vi "Set Label Config.vi"(8 "error in (no error)":errorcluster, 11 "RT Data in":T1 {"Label Transfer Config"."Block Data Refs"."Data Reference" format="%.0x"; "Status Config"."HWOut Dur Ref" format="%.0x"; "Status Config"."HWIn Dur Ref" format="%.0x"; "Status Config"."Error Data Ref" format="%.0x"; "HWOutput Channels"."Labels Settings"."Label" format="%.0o"; "HWInput Channels"."Labels Settings"."Label" format="%.0o"}) -> (0 "error out":errorcluster, 3 "RT Data out":T1 {"Label Transfer Config"."Block Data Refs"."Data Reference" format="%.0x"; "Status Config"."HWOut Dur Ref" format="%.0x"; "Status Config"."HWIn Dur Ref" format="%.0x"; "Status Config"."Error Data Ref" format="%.0x"; "HWOutput Channels"."Labels Settings"."Label" format="%.0o"; "HWInput Channels"."Labels Settings"."Label" format="%.0o"})   [LabVIEW 2015, in "AIT 429 Engine.lvlib"]
uses:
  AIT 429 Engine.lvlib
  RT Controls/RT Data.ctl
  RT Controls/RT HW Channel.ctl
  RT Controls/RT Label Settings.ctl
  Shared/Controls and Global/Label.ctl
  Shared/Controls and Global/transferPeriod.ctl
  RT Controls/Driver Data.ctl
  RT Controls/RT Word Settings.ctl
  <vilib>/NI Veristand/Custom Device API/Block Data Reference.ctl
  <vilib>/NI Veristand/Custom Device API/Data Reference.ctl
  RT Controls/RT Param Setting.ctl
  Shared/Controls and Global/Start Bit.ctl
  Shared/Controls and Global/Number of Bits.ctl
  Shared/Controls and Global/TransferType.ctl
  RT Controls/Error Qs.ctl
  RT Controls/Status Channels Config.ctl
  RT Controls/FIFO.ctl
  RT Controls/Label Transfer Config.ctl
  <instrlib>/AIT 429/AIT 429.lvlib
  Shared/AIT 429 Shared.lvlib
  <vilib>/NI Veristand/Custom Device API/Custom Device API.lvlib
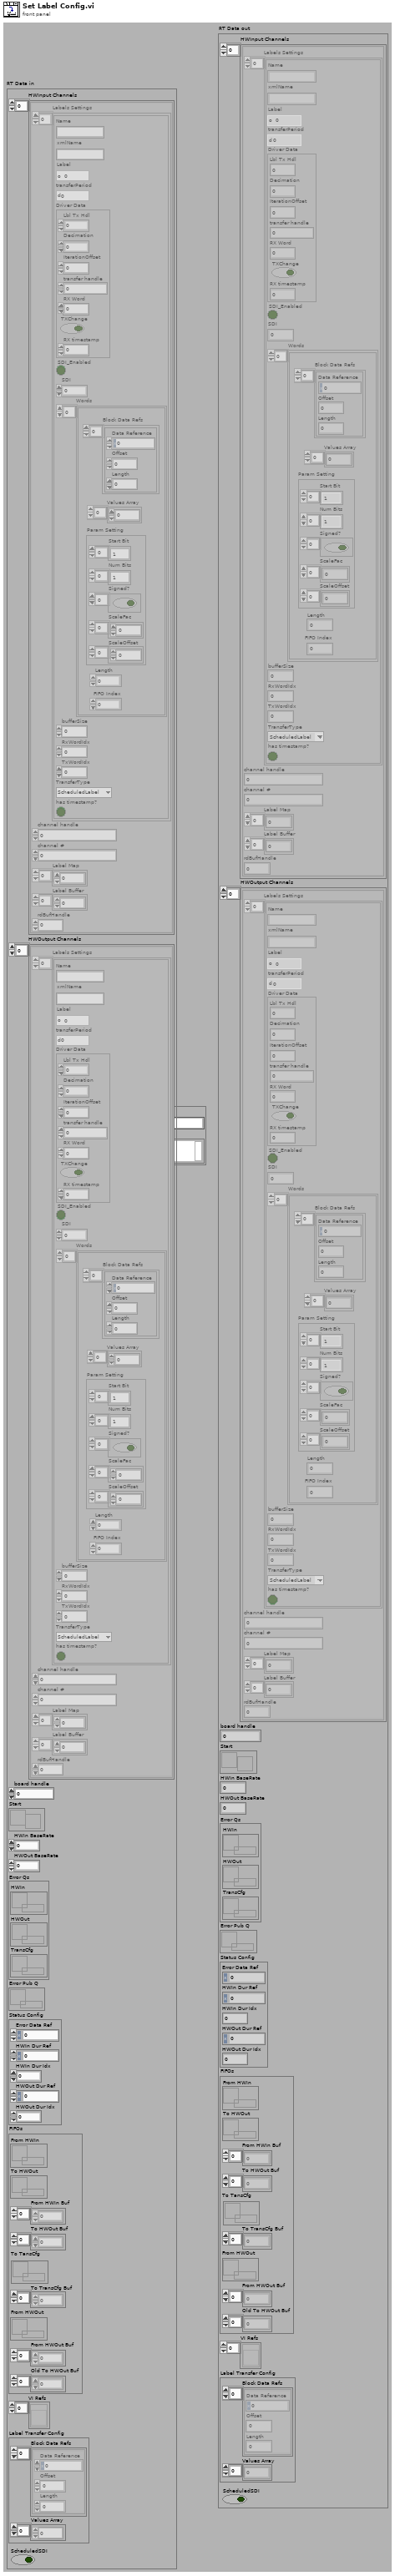
[diagram p1: front panel]
types:
  T1 = typedef "AIT 429 Engine.lvlib/RT Data.ctl" = cluster{"HWInput Channels":T2[], "HWOutput Channels":T2[], "board handle":u32, "Start":refnum<notifier>, "HWIn BaseRate":i64, "HWOut BaseRate":i64, "Error Qs":T14, "Error Pub Q":refnum<queue>, "Status Config":T15, "FIFOs":T16, "VI Refs":refnum<vi>[], "Label Transfer Config":T17, "ScheduledSDI":bool}
  T2 = typedef "AIT 429 Engine.lvlib/RT HW Channel.ctl" = cluster{"Labels Settings":T3[], "channel handle":u32, "channel #":u16, "Label Map":i32[], "Label Buffer":u32[], "rdBufHandle":u32}
  T3 = typedef "AIT 429 Engine.lvlib/RT Label Settings.ctl" = cluster{"Name":string, "xmlName":string, "Label":T4, "transferPeriod":T5, "Driver Data":T6, "SDI_Enabled":bool, "SDI":u8, "Words":T7[], "bufferSize":u32, "RxWordIdx":i32, "TxWordIdx":i32, "TransferType":T13, "has timestamp?":bool}
  T4 = typedef "AIT 429 Shared.lvlib/Label.ctl" = u8
  T5 = typedef "AIT 429 Shared.lvlib/transferPeriod.ctl" = u32
  T6 = typedef "AIT 429 Engine.lvlib/Driver Data.ctl" = cluster{"Lbl Tx Hdl":u32, "Decimation":i32, "IterationOffset":i32, "transfer handle":u32, "RX Word":u32, "TXChange":bool, "RX timestamp":dbl}
  T7 = typedef "AIT 429 Engine.lvlib/RT Word Settings.ctl" = cluster{"Block Data Refs":T8[], "Values Array":dbl[], "Length":i32, "FIFO Index":i32, "Param Setting":T10}
  T8 = typedef "Custom Device API.lvlib/Block Data Reference.ctl" = cluster{"Data Reference":T9, "Offset":u64, "Length":u64}
  T9 = typedef "Custom Device API.lvlib/Data Reference.ctl" = i32
  T10 = typedef "AIT 429 Engine.lvlib/RT Param Setting.ctl" = cluster{"Start Bit":T11[], "Num Bits":T12[], "Signed?":bool[], "ScaleFac":dbl[], "ScaleOffset":dbl[]}
  T11 = typedef "AIT 429 Shared.lvlib/Start Bit.ctl" = i32
  T12 = typedef "AIT 429 Shared.lvlib/Number of Bits.ctl" = i32
  T13 = typedef "AIT 429 Shared.lvlib/TransferType.ctl" = enum16{"ScheduledLabel", "Acyclic", "Block", "Strobe"}
  T14 = typedef "AIT 429 Engine.lvlib/Error Qs.ctl" = cluster{"HWIn":refnum<queue>, "HWOut":refnum<queue>, "TransCfg":refnum<queue>}
  T15 = typedef "AIT 429 Engine.lvlib/Status Channels Config.ctl" = cluster{"Error Data Ref":T9, "HWIn Dur Ref":T9, "HWIn Dur Idx":i32, "HWOut Dur Ref":T9, "HWOut Dur Idx":i32}
  T16 = typedef "AIT 429 Engine.lvlib/FIFO.ctl" = cluster{"From HWIn":refnum<k33>, "To HWOut":refnum<k33>, "From HWIn Buf":dbl[], "To HWOut Buf":dbl[], "To TansCfg":refnum<k33>, "To TransCfg Buf":dbl[], "From HWOut":refnum<k33>, "From HWOut Buf":dbl[], "Old To HWOut Buf":dbl[]}
  T17 = typedef "AIT 429 Engine.lvlib/Label Transfer Config.ctl" = cluster{"Block Data Refs":T8[], "Values Array":dbl[]}
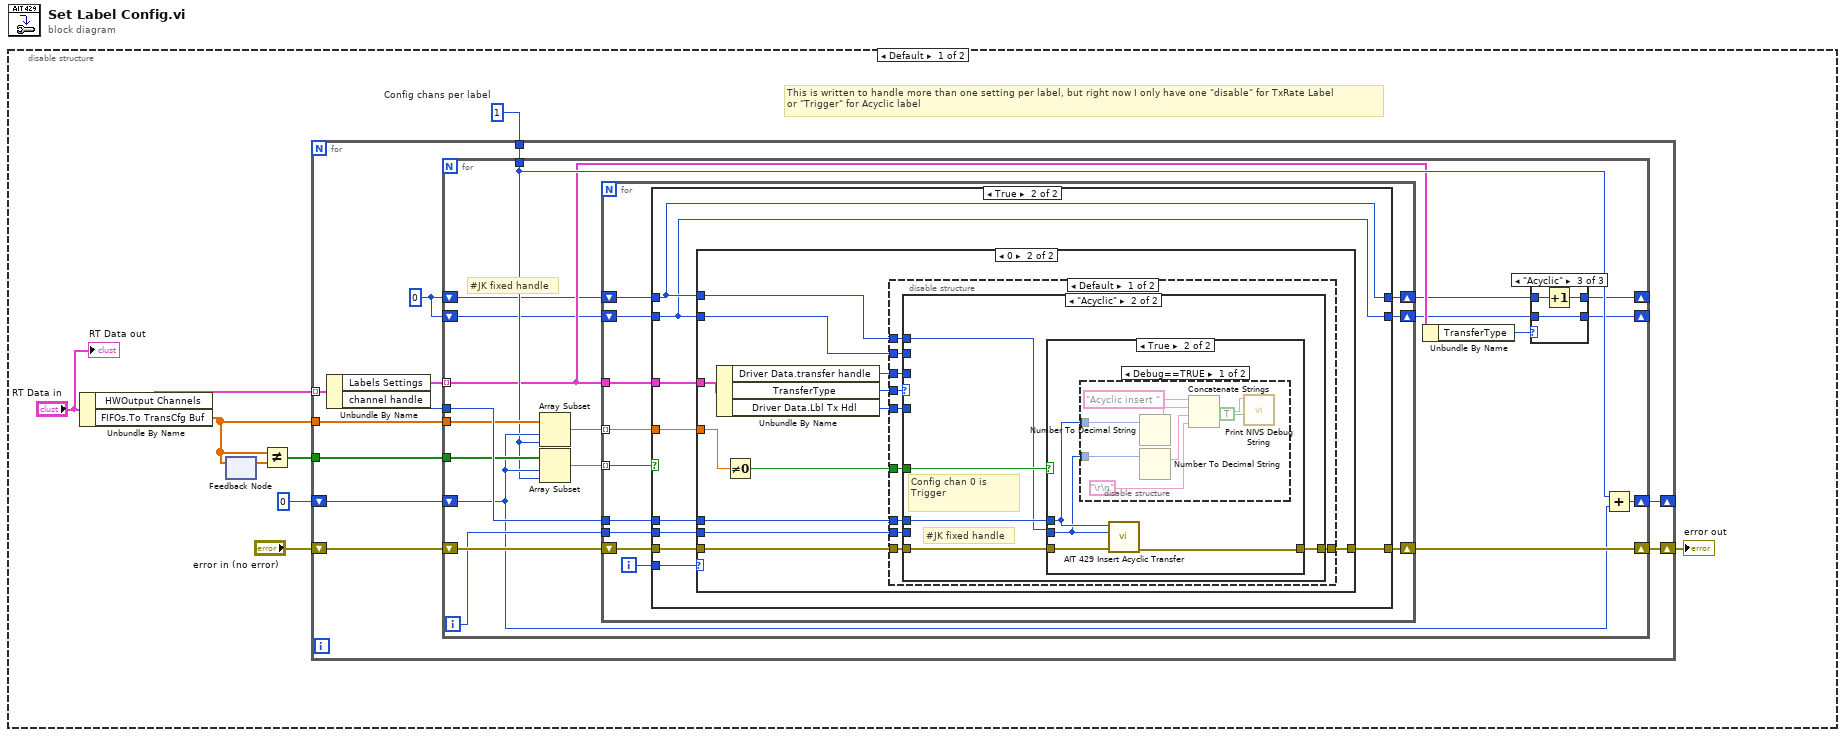
[diagram p0: block diagram]
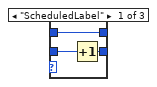
[diagram p2: hidden frame]
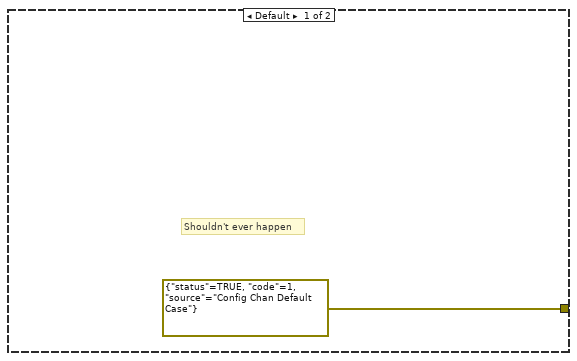
[diagram p5: hidden frame]
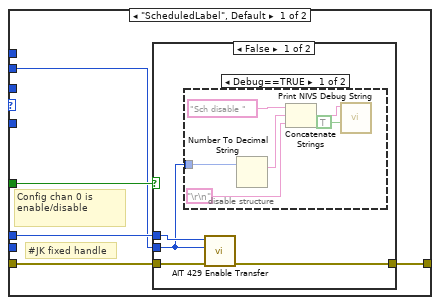
[diagram p6: hidden frame]
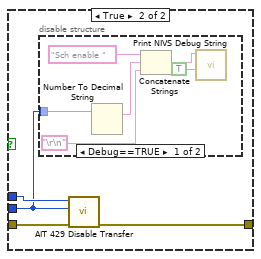
[diagram p8: hidden frame]
diagram:
  n1 = disable-structure shown="Default" {
    frame condition #0 (active) {
      w2 = 1  # Config chans per label
      # "This is written to handle more than one setting per label, but right now I only have one \"disable\" for TxRate Label \nor \"Trigger\" for Acyclic label"
      n2 = Unbundle By Name("RT Data in") -> ("HWOutput Channels"=w7:T2[], "FIFOs.To TransCfg Buf"=w1:dbl[])
      n3 = feedback #1() -> (w5:dbl[])  [unwired: 1 in]
      n4 = feedback-in #1(w1) -> ()
      n5 = Not Equal?(x=w1, y=w5) -> (x != y?=w4:bool[])
      n6 = for {
        shift-right: [w19] -> w8
        shift-left: "error in (no error)" -> [w20]
        tunnel: w7 -> [w18] mode=indexing
        shift-right: [w12] -> _
        shift-left: 0 ("index") -> [w14]
        tunnel: w4 -> [w15]
        tunnel: w2 -> [w13]
        tunnel: w1 -> [w11]
        w10 = u32 0 ("Lbl Tx Hdl")
        n7 = Unbundle By Name(w18) -> ("Labels Settings"=w17:T3[], "channel handle"=w16:u32)
        n8 = for {
          tunnel: w17 -> [w25] mode=indexing
          tunnel: w16 -> [w37]
          shift-right: [w38] -> w19
          shift-left: w20 -> [w39]
          tunnel: w15 -> [w36]
          tunnel: w13 -> [w30]
          shift-right: [w34] -> w12
          shift-left: w14 -> [w31]
          tunnel: w11 -> [w32]
          shift-right: [w27] -> _
          shift-left: w10 -> [w22]
          shift-right: [w26] -> _
          shift-left: w10 -> [w21]
          i -> [w33]
          # "#JK fixed handle"
          n9 = Array Subset(array=w32, index=w31, length=w30) -> (w29:dbl[])
          n10 = Array Subset(array=w36, index=w31, length=w30) -> (w35:bool[])
          n11 = for {
            tunnel: w37 -> [w57]
            tunnel: w35 -> [w55] mode=indexing
            tunnel: w33 -> [w56]
            shift-right: [w58] -> w38
            shift-left: w39 -> [w59]
            tunnel: w29 -> [w54] mode=indexing
            tunnel: w25 -> [w50]
            shift-right: [w51] -> w23
            shift-left: w21 -> [w48]
            shift-right: [w52] -> w24
            shift-left: w22 -> [w49]
            i -> [w53]
            n12 = case shown="True" w55 {
              tunnel: w59 -> [w62 w71]
              tunnel: [w62 w70] -> w58
              tunnel: w57 -> [_ w69]
              tunnel: w56 -> [_ w68]
              tunnel: w54 -> [_ w66]
              tunnel: w53 -> [_ w67]
              tunnel: w50 -> [_ w65]
              tunnel: [w61 w64] -> w52
              tunnel: [w60 w63] -> w51
              tunnel: w49 -> [w61 w64]
              tunnel: w48 -> [w60 w63]
              frame False {
              }
              frame True {
                n13 = case shown="0" w67 {
                  tunnel: w71 -> [_ w84]
                  tunnel: [errorcluster {"status"=TRUE, "code"=1, "source"="Config Chan Default Case"} ("error out") w83] -> w70
                  tunnel: w69 -> [_ w82]
                  tunnel: w68 -> [_ w81]
                  tunnel: w66 -> [_ w80]
                  tunnel: w65 -> [_ w78]
                  tunnel: w64 -> [_ w74]
                  tunnel: w63 -> [_ w73]
                  frame Default {
                    # "Shouldn't ever happen"
                  }
                  frame 0 {
                    n14 = Unbundle By Name(w78) -> ("Driver Data.transfer handle"=w76:u32, "TransferType"=w77:T13, "Driver Data.Lbl Tx Hdl"=w75:u32)
                    n15 = Not Equal To 0?(x=w80) -> (x != 0?=w79:bool)
                    n16 = disable-structure shown="Default" {
                      disable-tunnel: w84 -> [w94 w138]
                      disable-tunnel: [w93 w138] -> w83
                      disable-tunnel: w82 -> [w92 _]
                      disable-tunnel: w81 -> [w91 _]
                      disable-tunnel: w79 -> [w90 _]
                      disable-tunnel: w77 -> [w89 _]
                      disable-tunnel: w76 -> [w88 _]
                      disable-tunnel: w75 -> [w87 _]
                      disable-tunnel: w74 -> [w86 _]
                      disable-tunnel: w73 -> [w85 _]
                      frame condition #0 (active) {
                        n17 = case shown="\"Acyclic\"" w89 {
                          tunnel: w94 -> [w99 w124]
                          tunnel: [w98 w123] -> w93
                          tunnel: w92 -> [w97 w122]
                          tunnel: w91 -> [_ _]
                          tunnel: w90 -> [w96 w121]
                          tunnel: w88 -> [_ _]
                          tunnel: w87 -> [_ _]
                          tunnel: w86 -> [_ w120]
                          tunnel: w85 -> [w95 _]
                          frame "ScheduledLabel", Default {
                            # "#JK fixed handle"
                            # "Config chan 0 is enable/disable"
                            n18 = case shown="False" w96 {
                              tunnel: w99 -> [w102 w113]
                              tunnel: [w103 w112] -> w98
                              tunnel: w97 -> [w101 w111]
                              tunnel: w95 -> [w100 w110]
                              frame False {
                                n19 = disable-structure shown="Debug==TRUE" {
                                disable-tunnel: w100 -> [w107 _]
                                frame condition #0 {
                                n20 = Number To Decimal String(number=w107) -> (decimal integer string=w106:string)  [unwired: 1 in]
                                n21 = Concatenate Strings("Sch disable ", w106, "\r\n") -> (w108:string)
                                n22 = call "Print NIVS Debug String.vi"("Add to NIVS Log FIle? (T)"=TRUE, "Debug String"=w108) -> ()  [unwired: 8 in, 1 out]
                                }
                                frame condition #1 (active) {
                                }
                                }
                                n23 = call <instrlib>:"AIT 429 Enable Transfer.vi"("error in (no error)"=w102, "transfer handle in"=w100, "Tx channel handle in"=w101) -> ("error out"=w103:errorcluster)  [unwired: 7 in, 1 out]
                              }
                              frame True {
                                n24 = disable-structure shown="Debug==TRUE" {
                                disable-tunnel: w110 -> [w116 _]
                                frame condition #0 {
                                n25 = Number To Decimal String(number=w116) -> (decimal integer string=w115:string)  [unwired: 1 in]
                                n26 = Concatenate Strings("Sch enable ", w115, "\r\n") -> (w117:string)
                                n27 = call "Print NIVS Debug String.vi"("Add to NIVS Log FIle? (T)"=TRUE, "Debug String"=w117) -> ()  [unwired: 8 in, 1 out]
                                }
                                frame condition #1 (active) {
                                }
                                }
                                n28 = call <instrlib>:"AIT 429 Disable Transfer.vi"("error in"=w113, "transfer handle in"=w110, "Tx channel handle in"=w111) -> ("error out"=w112:errorcluster)  [unwired: 6 in, 2 out]
                              }
                            }
                          }
                          frame "Acyclic" {
                            # "#JK fixed handle"
                            # "Config chan 0 is \nTrigger"
                            n29 = case shown="True" w121 {
                              tunnel: w124 -> [w125 w129]
                              tunnel: [w125 w128] -> w123
                              tunnel: w122 -> [_ w127]
                              tunnel: w120 -> [_ w126]
                              frame False {
                              }
                              frame True {
                                n30 = disable-structure shown="Debug==TRUE" {
                                disable-tunnel: w126 -> [w134 _]
                                disable-tunnel: w127 -> [w131 _]
                                frame condition #0 {
                                n31 = Number To Decimal String(number=w131) -> (decimal integer string=w130:string)  [unwired: 1 in]
                                n32 = Number To Decimal String(number=w134) -> (decimal integer string=w133:string)  [unwired: 1 in]
                                n33 = Concatenate Strings("Acyclic insert ", w130, w133, "\r\n") -> (w135:string)
                                n34 = call "Print NIVS Debug String.vi"("Add to NIVS Log FIle? (T)"=TRUE, "Debug String"=w135) -> ()  [unwired: 8 in, 1 out]
                                }
                                frame condition #1 (active) {
                                }
                                }
                                n35 = call <instrlib>:"AIT 429 Insert Acyclic Transfer.vi"("error in (no error)"=w129, "acyclic handle"=w126, "channel handle"=w127) -> ("error out"=w128:errorcluster)  [unwired: 7 in, 1 out]
                              }
                            }
                          }
                        }
                      }
                      frame condition #1 {
                      }
                    }
                  }
                }
              }
            }
          }
          n36 = Unbundle By Name(w25) -> ("TransferType"=w28:T13)
          n37 = case shown="\"Acyclic\"" w28 {
            tunnel: w24 -> [w41 w44 w47]
            tunnel: w23 -> [w42 w43 w45]
            tunnel: [w41 w44 w46] -> w27
            tunnel: [w40 w43 w45] -> w26
            frame "ScheduledLabel" {
              n38 = Increment(x=w42) -> (x+1=w40:u32)
            }
            frame "Block", Default {
            }
            frame "Acyclic" {
              n39 = Increment(x=w47) -> (x+1=w46:u32)
            }
          }
          n40 = Add(x=w30, y=w31) -> (x+y=w34:i32)
        }
      }
      "error out" <- w8
      "RT Data out" <- "RT Data in"
    }
    frame condition #1 {
      # "writing not implemented"
    }
  }
